vi "Configure Frequency Array Scan.vi"(8 "error in (no error)":errorcluster, 10 "frequencies, Hz":u32[](array[numeric]), 11 "VI Probe in":refnum<class "PL MKS VI Probe.lvclass">) -> (0 "error out":errorcluster, 3 "VI Probe out":refnum<class "PL MKS VI Probe.lvclass">)   [LabVIEW 2015, in "PL MKS VI Probe.lvclass"]
doc: "Configures frequency scan, specified by the array of frequencies."
uses:
  PL MKS VI Probe.lvclass
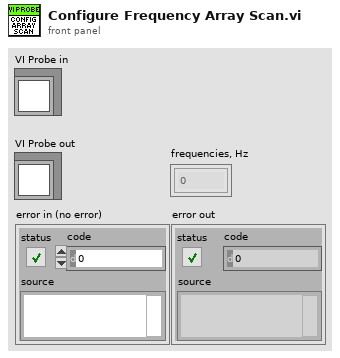
[diagram p1: front panel]
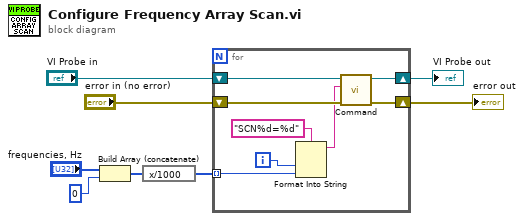
[diagram p0: block diagram]
diagram:
  n1 = Build Array (concatenate)("frequencies, Hz", u32 0 ("Numeric")) -> (w2:u32[])
  n2 = expression code="x/1000"(w2) -> (w1:u32[])
  n3 = for {
    shift-right: [w13] -> w6
    shift-left: "VI Probe in" -> [w15]
    shift-right: [w12] -> w5
    shift-left: "error in (no error)" -> [w14]
    tunnel: w1 -> [w10] mode=indexing
    i -> [w9]
    n4 = Format Into String(format string="SCN%d=%d", w9, w10) -> (resulting string=w11:string)  [unwired: 2 in, 1 out]
    n5 = call "Command.vi"("error in (no error)"=w14, "command"=w11, "VI Probe in"=w15) -> ("error out"=w12:errorcluster, "VI Probe out"=w13:refnum<class "PL MKS VI Probe.lvclass">)  [unwired: 6 in, 1 out]
  }
  "VI Probe out" <- w6
  "error out" <- w5
